vi "CRYUpdate Unicode Tab Pages.vi"(5 "Interpret as Unicode (T)":bool=TRUE, 6 "error in":errorcluster, 7 "Page Captions":string[](array[string]), 9 "Tab Control":refnum<vi>) -> (0 "error out":errorcluster, 3 "Tab Control":refnum<vi>)   [LabVIEW 2013]
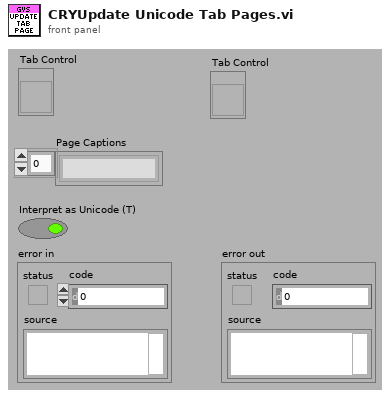
[diagram p1: front panel]
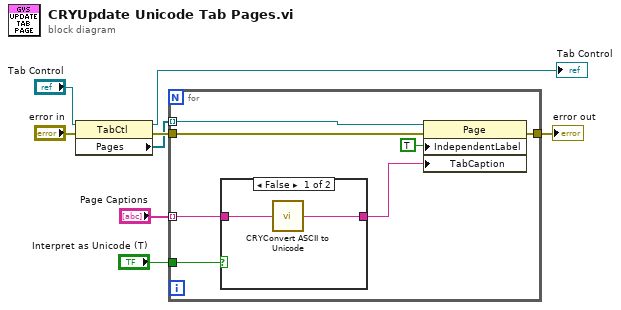
[diagram p0: block diagram]
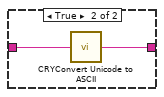
[diagram p2: hidden frame]
diagram:
  n1 = property class="TabCtl"(reference="Tab Control", error in="error in") -> (reference out=→"Tab Control":refnum<vi>, error out=w6:errorcluster, "Pages"=w5:refnum<vi>[])
  n2 = for {
    tunnel: w5 -> [w10] mode=indexing
    tunnel: w6 -> [w15]
    tunnel: "Page Captions" -> [w11] mode=indexing
    tunnel: [w13] -> w8
    tunnel: "Interpret as Unicode (T)" -> [w12]
    n3 = case shown="False" w12 {
      tunnel: [w16 w18] -> w9
      tunnel: w11 -> [w17 w19]
      frame False {
        n4 = call "CRYConvert ASCII to Unicode.vi"("ASCII"=w17) -> ("Unicode"=w16:string)  [unwired: 4 in]
      }
      frame True {
        n5 = call "CRYConvert Unicode to ASCII.vi"("Unicode"=w19) -> ("ASCII"=w18:string)  [unwired: 4 in]
      }
    }
    n6 = property class="Page"(reference=w10, error in=w15, "IndependentLabel"=TRUE ("Independent Label"), "TabCaption"=w9) -> (error out=w13:errorcluster)  [unwired: 1 out]
  }
  "error out" <- w8
